vi "LoggerHelper-MotorControllers.vi"(10 "Talon SRX Status Input":T1, 11 "Prefix Name":string) -> (2 "Talon Log Data":string)   [LabVIEW 2014]
uses:
  <vilib>/Rock Robotics/WPI/CAN/TalonSRX/WPI_CANTalonSRX_GlobalStatus.ctl
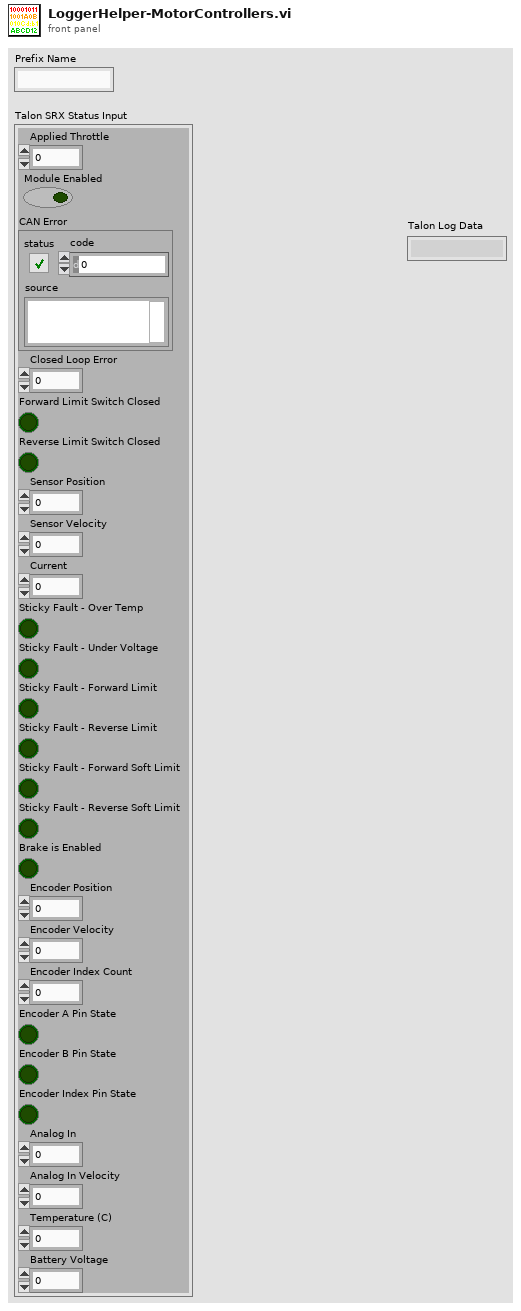
[diagram p1: front panel]
types:
  T1 = typedef "WPI_CANTalonSRX_GlobalStatus.ctl" = cluster{"Applied Throttle":dbl, "Module Enabled":bool, "CAN Error":errorcluster, "Closed Loop Error":dbl, "Forward Limit Switch Closed":bool, "Reverse Limit Switch Closed":bool, "Sensor Position":dbl, "Sensor Velocity":dbl, "Current":dbl, "Sticky Fault - Over Temp":bool, "Sticky Fault - Under Voltage":bool, "Sticky Fault - Forward Limit":bool, "Sticky Fault - Reverse Limit":bool, "Sticky Fault - Forward Soft Limit":bool, "Sticky Fault - Reverse Soft Limit":bool, "Brake is Enabled":bool, "Encoder Position":dbl, "Encoder Velocity":dbl, "Encoder Index Count":dbl, "Encoder A Pin State":bool, "Encoder B Pin State":bool, "Encoder Index Pin State":bool, "Analog In":dbl, "Analog In Velocity":dbl, "Temperature (C)":dbl, "Battery Voltage":dbl}
  T2 = cluster{"Applied Throttle":bool, "Module Enabled":bool, "CAN Error":cluster{"status":bool, "code":bool, "source":bool}, "Closed Loop Error":bool, "Forward Limit Switch Closed":bool, "Reverse Limit Switch Closed":bool, "Sensor Position":bool, "Sensor Velocity":bool, "Current":bool, "Sticky Fault - Over Temp":bool, "Sticky Fault - Under Voltage":bool, "Sticky Fault - Forward Limit":bool, "Sticky Fault - Reverse Limit":bool, "Sticky Fault - Forward Soft Limit":bool, "Sticky Fault - Reverse Soft Limit":bool, "Brake is Enabled":bool, "Encoder Position":bool, "Encoder Velocity":bool, "Encoder Index Count":bool, "Encoder A Pin State":bool, "Encoder B Pin State":bool, "Encoder Index Pin State":bool, "Analog In":bool, "Analog In Velocity":bool, "Temperature (C)":bool, "Battery Voltage":bool}
  T3 = cluster{"status":bool, "code":bool, "source":bool}
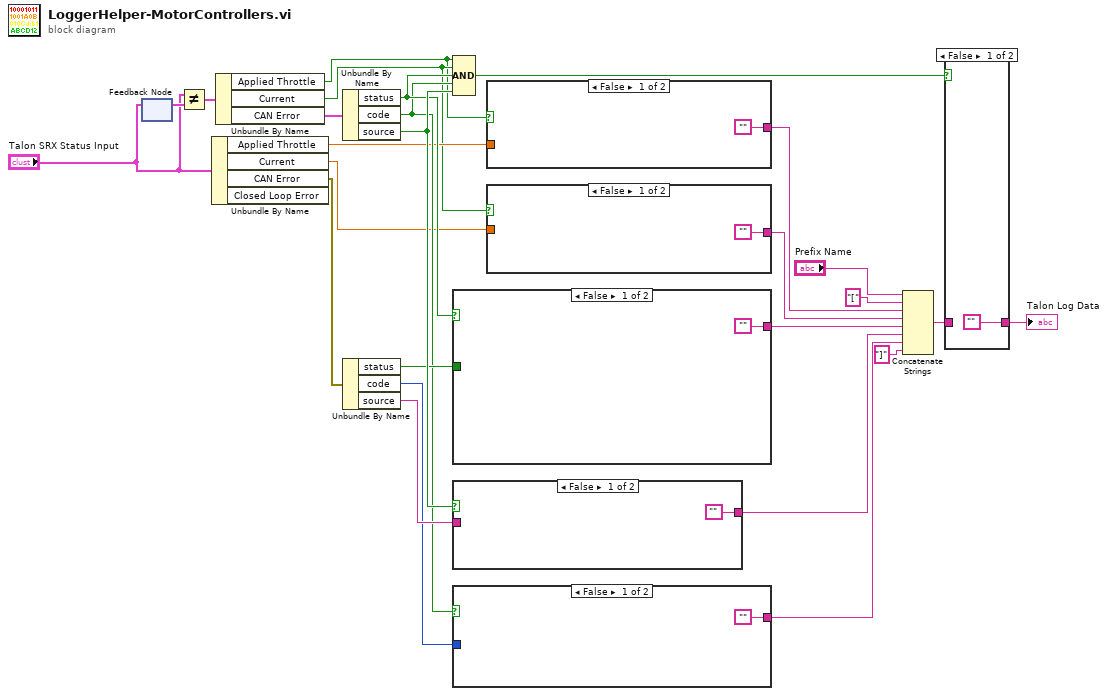
[diagram p0: block diagram]
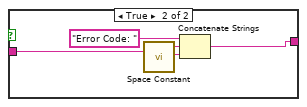
[diagram p3: hidden frame]
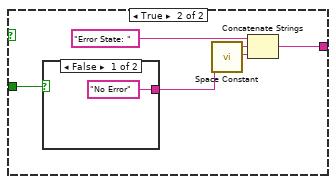
[diagram p4: hidden frame]
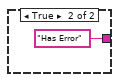
[diagram p5: hidden frame]
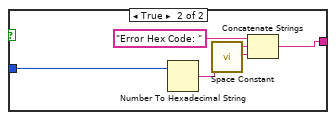
[diagram p6: hidden frame]
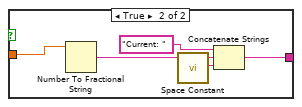
[diagram p7: hidden frame]
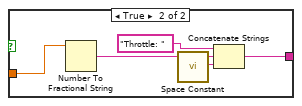
[diagram p8: hidden frame]
diagram:
  n1 = feedback #1() -> (w12:T1)  [unwired: 1 in]
  n2 = feedback-in #1("Talon SRX Status Input") -> ()
  n3 = Not Equal?(x="Talon SRX Status Input", y=w12) -> (x != y?=w13:T2)
  n4 = Unbundle By Name("Talon SRX Status Input") -> ("Applied Throttle"=w19:dbl, "Current"=w18:dbl, "CAN Error"=w15:errorcluster)  [unwired: 1 out]
  n5 = Unbundle By Name(w13) -> ("Applied Throttle"=w16:bool, "Current"=w17:bool, "CAN Error"=w14:T3)
  n6 = Unbundle By Name(w14) -> ("status"=w22:bool, "code"=w21:bool, "source"=w24:bool)
  n7 = Unbundle By Name(w15) -> ("status"=w23:bool, "code"=w20:i32, "source"=w25:string)
  n8 = Compound Arithmetic op=AND(w16, w17, w22, w21, w24) -> (w11:bool)
  n9 = case shown="False" w22 {
    tunnel: w23 -> [_ w32]
    tunnel: ["" w31] -> w6
    frame False {
    }
    frame True {
      n10 = case shown="False" w32 {
        tunnel: ["No Error" "Has Error"] -> w30
        frame False {
        }
        frame True {
        }
      }
      n11 = call <vilib>:"Space Constant.vi"() -> ("String"=w28:string)
      n12 = Concatenate Strings("Error State: ", w30, w28) -> (w31:string)
    }
  }
  n13 = case shown="False" w24 {
    tunnel: w25 -> [_ w38]
    tunnel: ["" w39] -> w7
    frame False {
    }
    frame True {
      n14 = call <vilib>:"Space Constant.vi"() -> ("String"=w36:string)
      n15 = Concatenate Strings("Error Code: ", w38, w36) -> (w39:string)
    }
  }
  n16 = case shown="False" w21 {
    tunnel: w20 -> [_ w45]
    tunnel: ["" w42] -> w8
    frame False {
    }
    frame True {
      n17 = Number To Hexadecimal String(2:w45) -> (0:w44:string)  [unwired: 1 in]
      n18 = call <vilib>:"Space Constant.vi"() -> ("String"=w41:string)
      n19 = Concatenate Strings("Error Hex Code: ", w44, w41) -> (w42:string)
    }
  }
  n20 = case shown="False" w16 {
    tunnel: w19 -> [_ w51]
    tunnel: ["" w50] -> w4
    frame False {
    }
    frame True {
      n21 = Number To Fractional String(number=w51) -> (F-format string=w48:string)  [unwired: 3 in]
      n22 = call <vilib>:"Space Constant.vi"() -> ("String"=w47:string)
      n23 = Concatenate Strings("Throttle: ", w48, w47) -> (w50:string)
    }
  }
  n24 = case shown="False" w17 {
    tunnel: w18 -> [_ w57]
    tunnel: ["" w56] -> w5
    frame False {
    }
    frame True {
      n25 = Number To Fractional String(number=w57) -> (F-format string=w55:string)  [unwired: 3 in]
      n26 = call <vilib>:"Space Constant.vi"() -> ("String"=w53:string)
      n27 = Concatenate Strings("Current: ", w55, w53) -> (w56:string)
    }
  }
  n28 = Concatenate Strings("Prefix Name", "[", w4, w5, w6, w7, w8, "]") -> (w10:string)
  n29 = case shown="False" w11 {
    tunnel: w10 -> [_ w59]
    tunnel: ["" w59] -> w9
    frame False {
    }
    frame True {
    }
  }
  "Talon Log Data" <- w9
